vi "Rx.vi"(6 "Wait for? (\\r\\n)":string="\r\n", 7 "Timeout_ms (3000)":u32=3000, 8 "error in":errorcluster, 11 "VISA in":refnum<visa-resource-name>) -> (0 "error out":errorcluster, 1 "Response":string, 2 "Timeout?":bool, 3 "VISA out":refnum<visa-resource-name>, 5 "ExecTime(ms)":i32)   [LabVIEW 2016, in "Serial_G.lvlib"]
doc: "Read from VISA until \"Wait for\" string is found"
uses:
  Serial_G.lvlib
  <vilib>/regexp/Match Regular Expression.xnode
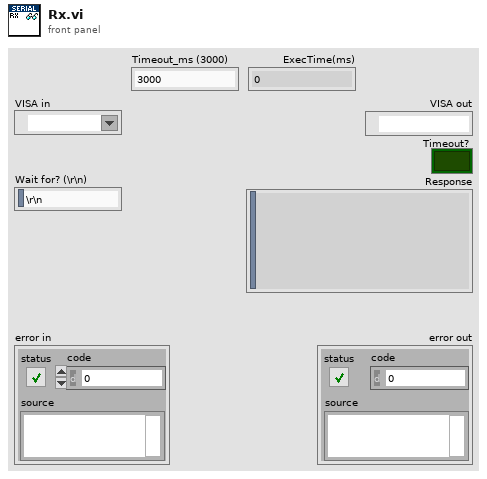
[diagram p1: front panel]
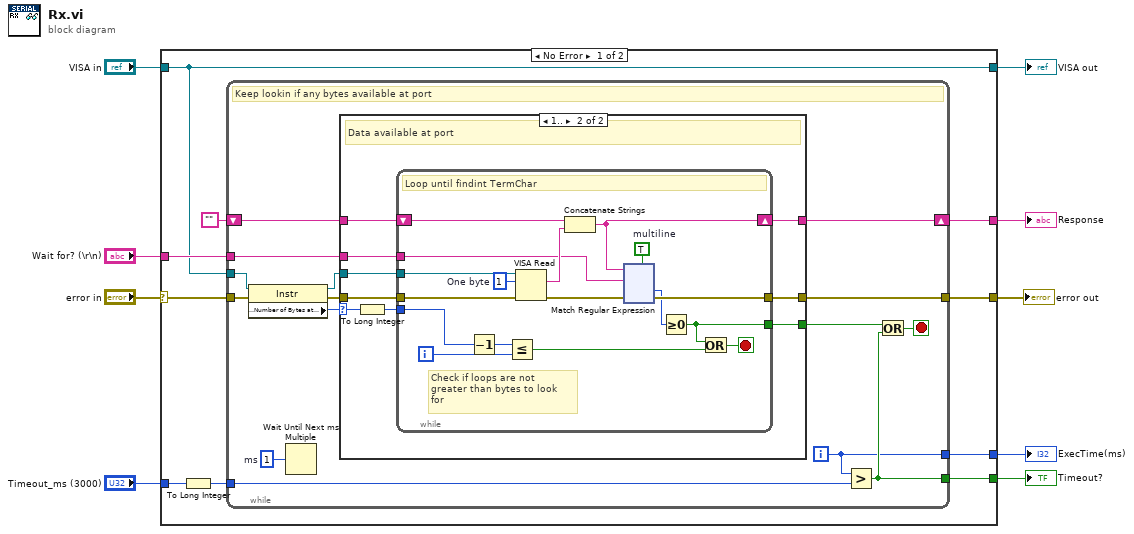
[diagram p0: block diagram]
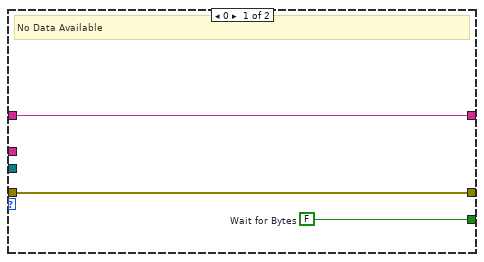
[diagram p2: hidden frame]
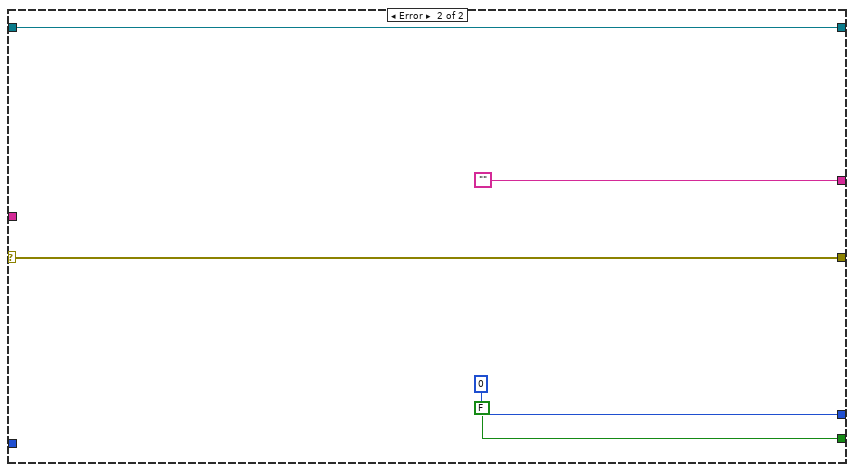
[diagram p3: hidden frame]
diagram:
  n1 = case shown="No Error" "error in" {
    selector: "error in" -> [w18 w182]
    tunnel: [w17 w182] -> w9
    tunnel: "VISA in" -> [w14 w179]
    tunnel: "Wait for? (\\r\\n)" -> [w16 _]
    tunnel: "Timeout_ms (3000)" -> [w15 _]
    tunnel: [w14 w179] -> w4
    tunnel: [w13 ""] -> w3
    tunnel: [w12 0] -> w2
    tunnel: [w11 FALSE] -> w1
    frame No Error {
      n2 = To Long Integer(number=w15) -> (32bit integer=w10:i32)
      n3 = while {
        tunnel: [w31] -> w17
        tunnel: w14 -> [w21]
        tunnel: w18 -> [w34]
        shift-right: [w30] -> w13
        shift-left: "" -> [w32]
        tunnel: [w27] -> w11
        tunnel: w16 -> [w24]
        tunnel: w10 -> [w23]
        tunnel: [w22] -> w12
        i -> [w22]
        stop <- w28 stop-if-true
        w29 = u32 1  # ms
        # "Keep lookin if any bytes available at port"
        n4 = property class="Instr"(reference=w21, error in=w34) -> (reference out=w20:refnum<visa-resource-name>, error out=w33:errorcluster, "Serial Settings:Number of Bytes at Serial Port"=w25:u32)
        n5 = Wait Until Next ms Multiple(millisecond multiple=w29) -> ()  [unwired: 1 out]
        n6 = case shown="1.." w25 {
          selector: w25 -> [_ w40]
          tunnel: w20 -> [_ w46]
          tunnel: w33 -> [w37 w45]
          tunnel: w32 -> [w36 w44]
          tunnel: [w37 w43] -> w31
          tunnel: [w36 w42] -> w30
          tunnel: [w35 w41] -> w26
          tunnel: w24 -> [_ w39]
          frame 0 {
            w35 = FALSE  # Wait for Bytes
            # "No Data Available"
          }
          frame 1.. {
            # "Data available at port"
            n7 = To Long Integer(number=w40) -> (32bit integer=w38:i32)
            n8 = while {
              tunnel: w46 -> [w62]
              tunnel: w45 -> [w61]
              tunnel: [w63] -> w43
              tunnel: [w54] -> w41
              shift-right: [w53] -> w42
              shift-left: w44 -> [w59]
              tunnel: w38 -> [w48]
              tunnel: w39 -> [w50]
              i -> [w49]
              stop <- w55 stop-if-true
              w47 = u32 1  # One byte
              w52 = TRUE  # multiline
              # "Check if loops are not \ngreater than bytes to look\nfor"
              # "Loop until findint TermChar"
              n9 = Decrement(x=w48) -> (x-1=w57:i32)
              n10 = Less Or Equal?(x=w57, y=w49) -> (x <= y?=w56:bool)
              n11 = VISA Read(VISA resource name=w62, byte count=w47, error in (no error)=w61) -> (read buffer=w58:string, error out=w51:errorcluster)  [unwired: 2 out]
              n12 = Concatenate Strings(w59, w58) -> (w53:string)
              n13 = xnode "Match Regular Expression"("input string"=w53, "regular expression"=w50, "error in"=w51, "multiline? (F)"=w52) -> ("offset past match"=w60:i32, "error out"=w63:errorcluster)  [unwired: 2 in, 3 out]
              n14 = Greater Or Equal To 0?(x=w60) -> (x >= 0?=w54:bool)
              n15 = Or(x=w54, y=w56) -> (x .or. y?=w55:bool)
            }
          }
        }
        n16 = Greater?(x=w22, y=w23) -> (0:w27:bool)
        n17 = Or(x=w26, y=w27) -> (x .or. y?=w28:bool)
      }
    }
    frame Error {
    }
  }
  "error out" <- w9
  "Response" <- w3
  "Timeout?" <- w1
  "VISA out" <- w4
  "ExecTime(ms)" <- w2
